vi "SMO Public API - constant.vi"(8 "error in (no error)":errorcluster, 11 "Instrument.Aerotech":refnum<class "Instrument.Aerotech.lvclass">) -> (0 "error out":errorcluster, 2 "Commands":string[](array[string]), 3 "Instrument.Aerotech out":refnum<class "Instrument.Aerotech.lvclass">)   [LabVIEW 2016, in "Instrument.Aerotech.lvclass"]
uses:
  Instrument.Aerotech.lvclass
  Typedefs/Instrument.Aerotech.Commands.ctl
  <userlib>/LevyLab/Levylab Instruments/Instrument Types/Optical Delay Line/Instrument.OpticalDelayLine.lvclass
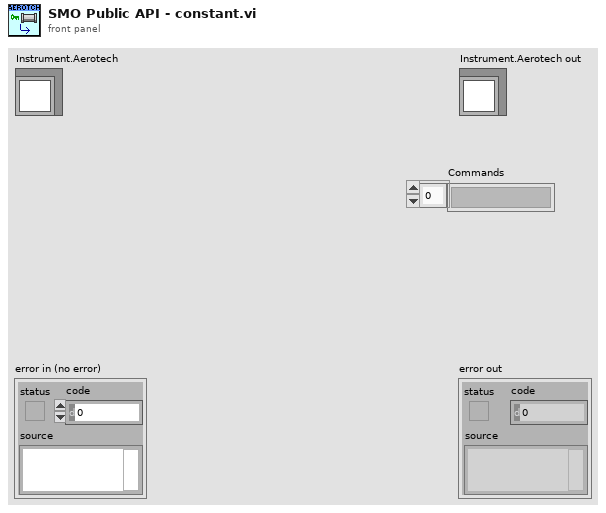
[diagram p1: front panel]
types:
  T1 = typedef "Instrument.Aerotech.lvclass/Instrument.Aerotech.Commands.ctl" = string[]
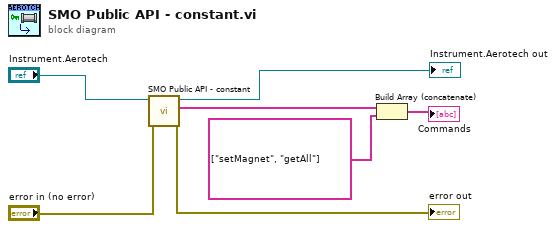
[diagram p0: block diagram]
diagram:
  n1 = call-parent "SMO Public API - constant.vi"("error in (no error)"="error in (no error)", "Instrument in"="Instrument.Aerotech") -> ("error out"=→"error out":errorcluster, "Commands"=w6:string[], "Instrument out"=→"Instrument.Aerotech out":refnum<class "Instrument.Aerotech.lvclass">)  [unwired: 7 in]
  n2 = Build Array (concatenate)(w6, T1 ["setMagnet", "getAll"] ("Array")) -> (→"Commands":T1)
